vi "SetFunction_XDM3051.vi"(8 "error in":errorcluster, 10 "Functions":T1, 11 "RS232_Input":refnum<visa-resource-name>) -> (0 "error out":errorcluster, 2 "response":string, 3 "RS232_Output":refnum<visa-resource-name>)   [LabVIEW 2017]
uses:
  controls/Functions_XDM3051.ctl
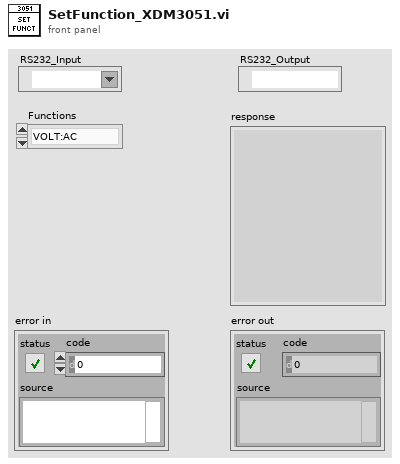
[diagram p1: front panel]
types:
  T1 = typedef "Functions_XDM3051.ctl" = enum16{"VOLT:AC", "VOLT:DC", "CURR:AC", "CURR:DC", "FREQ", "PER", "CAP", "CONT", "DIOD", "FRES", "RES", "TEMP:RTD"}
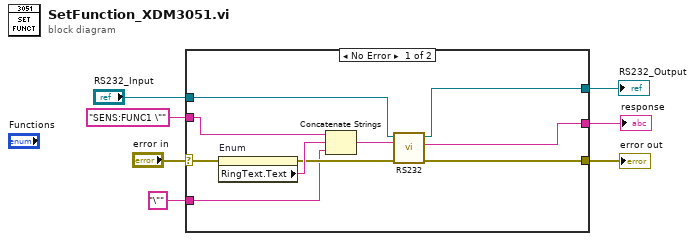
[diagram p0: block diagram]
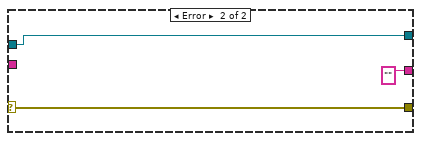
[diagram p2: hidden frame]
diagram:
  n1 = case shown="No Error" "error in" {
    selector: "error in" -> [w11 w20]
    tunnel: [w17 w20] -> w6
    tunnel: "RS232_Input" -> [w16 w19]
    tunnel: "SENS:FUNC1 \"" ("command") -> [w13 _]
    tunnel: [w15 "" ("response")] -> w3
    tunnel: [w14 w19] -> w2
    tunnel: "\"" ("command") -> [w9 _]
    frame No Error {
      n2 = property on="Enum" class="Enum (strict)"(error in=w11) -> (error out=w10:errorcluster, "RingText.Text"=w12:string)  [unwired: 1 in, 1 out]
      n3 = Concatenate Strings(w13, w12, w9) -> (w8:string)
      n4 = call "RS232.vi"("error in"=w10, "command"=w8, "RS232_Input"=w16) -> ("error out"=w17:errorcluster, "response"=w15:string, "RS232_Output"=w14:refnum<visa-resource-name>)  [unwired: 6 in]
    }
    frame Error {
    }
  }
  "error out" <- w6
  "RS232_Output" <- w2
  "response" <- w3
